vi "Remove VI.vi"(8 "error in (no error)":errorcluster, 10 "Index to remove":i32, 11 "Model in":refnum<class "Model.lvclass">) -> (0 "error out":errorcluster, 3 "Model out":refnum<class "Model.lvclass">)   [LabVIEW 2015, in "Model.lvlib" / "Model.lvclass"]
uses:
  Model.lvclass
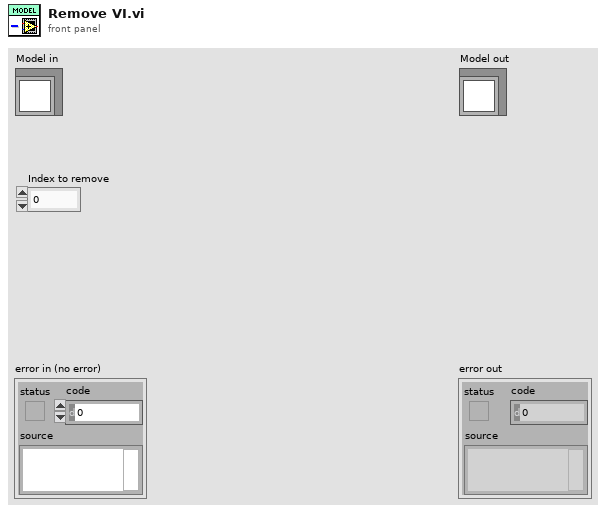
[diagram p1: front panel]
types:
  T1 = typedef "Model.lvlib/VI Infomation.ctl" = cluster{"Name":string, "Description":string, "Icon":picture}
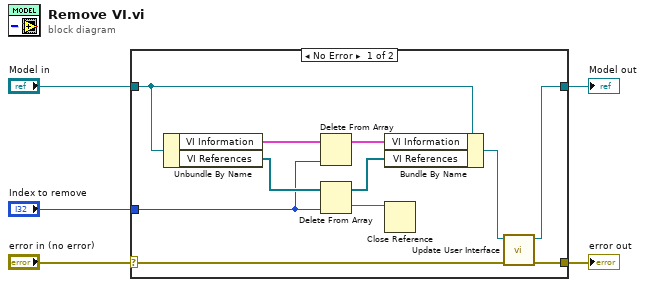
[diagram p0: block diagram]
diagram:
  n1 = case shown="No Error" "error in (no error)" {
    selector: "error in (no error)" -> [w7 w18]
    tunnel: [w6 w18] -> w4
    tunnel: [w8 w17] -> w2
    tunnel: "Model in" -> [w12 w17]
    tunnel: "Index to remove" -> [w13 _]
    frame No Error {
      n2 = Unbundle By Name(w12) -> ("VI Information"=w14:T1[], "VI References"=w16:refnum<vi>[])
      n3 = Delete From Array(array=w14, index=w13) -> (array with subset deleted=w11:T1[])  [unwired: 1 in, 1 out]
      n4 = Delete From Array(array=w16, index=w13) -> (deleted portion=w15:refnum<vi>, array with subset deleted=w10:refnum<vi>[])  [unwired: 1 in]
      n5 = Bundle By Name(cluster=w12, "VI Information"=w11, "VI References"=w10) -> (w9:refnum<class "Model.lvclass">)
      n6 = Close Reference(reference=w15) -> ()  [unwired: 1 in, 1 out]
      n7 = call "Update User Interface.vi"("error in (no error)"=w7, "Model in"=w9) -> ("error out"=w6:errorcluster, "Model out"=w8:refnum<class "Model.lvclass">)  [unwired: 8 in]
    }
    frame Error {
    }
  }
  "error out" <- w4
  "Model out" <- w2
